vi "超标留样流程.vi"   [LabVIEW 2016]
types:
  T1 = enum16{"德润DR803M", "德润DR803L", "德润DR803F", "科盛超标留样"}
  T2 = enum32{"Bad", "Idle", "Run top level", "Running"}
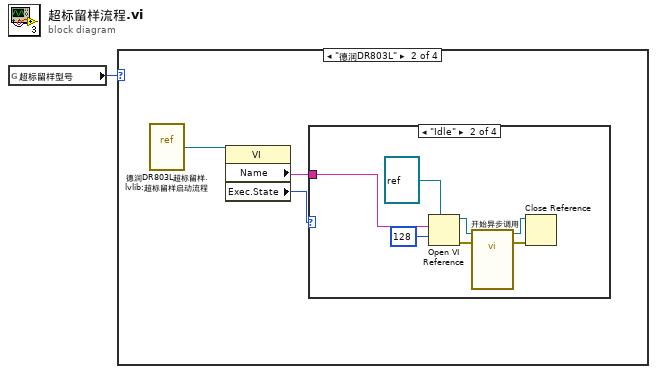
[diagram p0: block diagram]
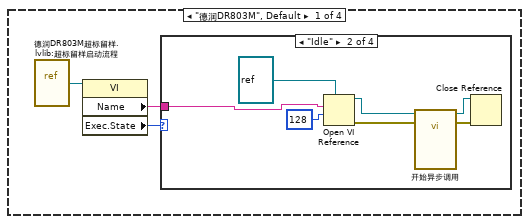
[diagram p2: hidden frame]
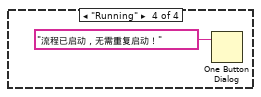
[diagram p5: hidden frame]
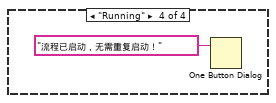
[diagram p8: hidden frame]
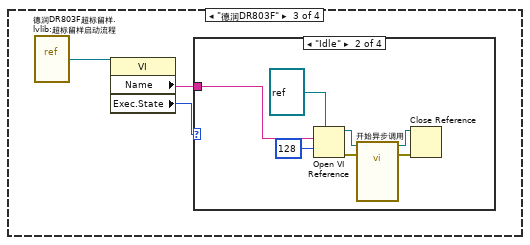
[diagram p9: hidden frame]
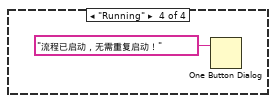
[diagram p12: hidden frame]
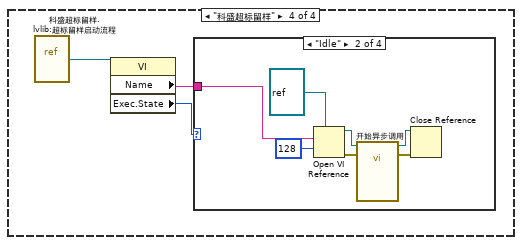
[diagram p13: hidden frame]
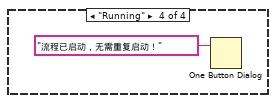
[diagram p16: hidden frame]
diagram:
  n1 = global read "断电保存全局.vi" "超标留样型号"() -> (w1:T1)
  n2 = case shown="\"德润DR803L\"" w1 {
    frame "德润DR803M", Default {
      n3 = vi-ref "德润DR803M超标留样.lvlib:超标留样启动流程.vi"() -> (w2:refnum<vi>)
      n4 = property class="VI"(reference=w2) -> ("Name"=w3:string, "Exec.State"=w4:T2)  [unwired: 1 in, 2 out]
      n5 = case shown="\"Idle\"" w4 {
        tunnel: w3 -> [_ w7 _ _]
        frame "Bad", Default {
        }
        frame "Idle" {
          n6 = Open VI Reference(type specifier VI Refnum (for type only)=refnum<vi> refnum ("类型说明符VI引用句柄（仅用于类型）"), vi path=w7, options=128 ("选项")) -> (vi reference=w11:refnum<vi>, error out=w6:errorcluster)  [unwired: 3 in]
          n7 = call-by-ref "开始异步调用"(reference=w11, error in=w6) -> (reference out=w10:refnum<vi>, error out=w5:errorcluster)  [unwired: 12 in]
          n8 = Close Reference(reference=w10, error in (no error)=w5) -> ()  [unwired: 1 out]
        }
        frame "Run top level" {
        }
        frame "Running" {
          n9 = One Button Dialog(message="流程已启动，无需重复启动！" ("消息")) -> ()  [unwired: 1 in, 1 out]
        }
      }
    }
    frame "德润DR803L" {
      n10 = vi-ref "德润DR803L超标留样.lvlib:超标留样启动流程.vi"() -> (w15:refnum<vi>)
      n11 = property class="VI"(reference=w15) -> ("Name"=w14:string, "Exec.State"=w13:T2)  [unwired: 1 in, 2 out]
      n12 = case shown="\"Idle\"" w13 {
        tunnel: w14 -> [_ w18 _ _]
        frame "Bad", Default {
        }
        frame "Idle" {
          n13 = Open VI Reference(type specifier VI Refnum (for type only)=refnum<vi> refnum ("类型说明符VI引用句柄（仅用于类型）"), vi path=w18, options=128 ("选项")) -> (vi reference=w22:refnum<vi>, error out=w17:errorcluster)  [unwired: 3 in]
          n14 = call-by-ref "开始异步调用"(reference=w22, error in=w17) -> (reference out=w21:refnum<vi>, error out=w16:errorcluster)  [unwired: 12 in]
          n15 = Close Reference(reference=w21, error in (no error)=w16) -> ()  [unwired: 1 out]
        }
        frame "Run top level" {
        }
        frame "Running" {
          n16 = One Button Dialog(message="流程已启动，无需重复启动！" ("消息")) -> ()  [unwired: 1 in, 1 out]
        }
      }
    }
    frame "德润DR803F" {
      n17 = vi-ref "德润DR803F超标留样.lvlib:超标留样启动流程.vi"() -> (w24:refnum<vi>)
      n18 = property class="VI"(reference=w24) -> ("Name"=w25:string, "Exec.State"=w26:T2)  [unwired: 1 in, 2 out]
      n19 = case shown="\"Idle\"" w26 {
        tunnel: w25 -> [_ w29 _ _]
        frame "Bad", Default {
        }
        frame "Idle" {
          n20 = Open VI Reference(type specifier VI Refnum (for type only)=refnum<vi> refnum ("类型说明符VI引用句柄（仅用于类型）"), vi path=w29, options=128 ("选项")) -> (vi reference=w33:refnum<vi>, error out=w28:errorcluster)  [unwired: 3 in]
          n21 = call-by-ref "开始异步调用"(reference=w33, error in=w28) -> (reference out=w32:refnum<vi>, error out=w27:errorcluster)  [unwired: 12 in]
          n22 = Close Reference(reference=w32, error in (no error)=w27) -> ()  [unwired: 1 out]
        }
        frame "Run top level" {
        }
        frame "Running" {
          n23 = One Button Dialog(message="流程已启动，无需重复启动！" ("消息")) -> ()  [unwired: 1 in, 1 out]
        }
      }
    }
    frame "科盛超标留样" {
      n24 = vi-ref "科盛超标留样.lvlib:超标留样启动流程.vi"() -> (w35:refnum<vi>)
      n25 = property class="VI"(reference=w35) -> ("Name"=w36:string, "Exec.State"=w37:T2)  [unwired: 1 in, 2 out]
      n26 = case shown="\"Idle\"" w37 {
        tunnel: w36 -> [_ w40 _ _]
        frame "Bad", Default {
        }
        frame "Idle" {
          n27 = Open VI Reference(type specifier VI Refnum (for type only)=refnum<vi> refnum ("类型说明符VI引用句柄（仅用于类型）"), vi path=w40, options=128 ("选项")) -> (vi reference=w44:refnum<vi>, error out=w39:errorcluster)  [unwired: 3 in]
          n28 = call-by-ref "开始异步调用"(reference=w44, error in=w39) -> (reference out=w43:refnum<vi>, error out=w38:errorcluster)  [unwired: 12 in]
          n29 = Close Reference(reference=w43, error in (no error)=w38) -> ()  [unwired: 1 out]
        }
        frame "Run top level" {
        }
        frame "Running" {
          n30 = One Button Dialog(message="流程已启动，无需重复启动！" ("消息")) -> ()  [unwired: 1 in, 1 out]
        }
      }
    }
  }
